vi "Ch_dis_to_Str_ADAM.vi"(4 "Ch Description":T1={"Ch Name"="", "Type"="", "Function"=enum."Analogue Input", "Ch State"=enum."On", "Calibration type"=enum."Raw", "A"=0.0, "B"=0.0, "C"=0.0, "D"=0.0, "Comments"="", "Address"={"Main"=0, "Ch."=0, "Sub"=0, "Port Name"=""}, "String"="", "Duty"=65535} {"Duty" format="%.0b"; "D" format="%#_5g"; "C" format="%#_5g"; "B" format="%#_5g"; "A" format="%#_5g"}) -> (1 "String Row":string)   [LabVIEW 2012]
uses:
  ADAM Controls/Ch_description_ADAM.ctl
  ADAM Controls/Module_type_ADAM.ctl
  ADAM Controls/Function_ADAM.ctl
  ADAM Controls/Channel_State.ctl
  ADAM Controls/Calib_type_ADAM.ctl
  ADAM Controls/Address.ctl
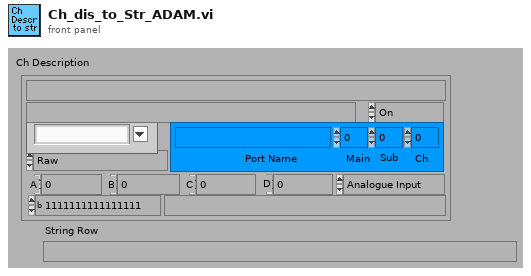
[diagram p1: front panel]
types:
  T1 = typedef "Ch_description_ADAM.ctl" = cluster{"Ch Name":string, "Type":T2, "Function":T3, "Ch State":T4, "Calibration type":T5, "A":dbl, "B":dbl, "C":dbl, "D":dbl, "Comments":string, "Address":T6, "String":string, "Duty":u16}
  T2 = typedef "Module_type_ADAM.ctl" = string
  T3 = typedef "Function_ADAM.ctl" = enum16{"Analogue Input", "Digital Input", "Event counter", "Event rate", "Analogue Output", "Digital Output", "Relay Output"}
  T4 = typedef "Channel_State.ctl" = enum16{"On", "Off", "Always On", "Always Off"}
  T5 = typedef "Calib_type_ADAM.ctl" = enum16{"Raw", "Bx + A", "Cx^2 + Bx + A", "Dx^3 + Cx^2 + Bx + A", "In Band", "Hi-Tec Q", "Hi-Tec M_dot", "Text"}
  T6 = typedef "Address.ctl" = cluster{"Main":i32, "Ch.":i32, "Sub":i32, "Port Name":string}
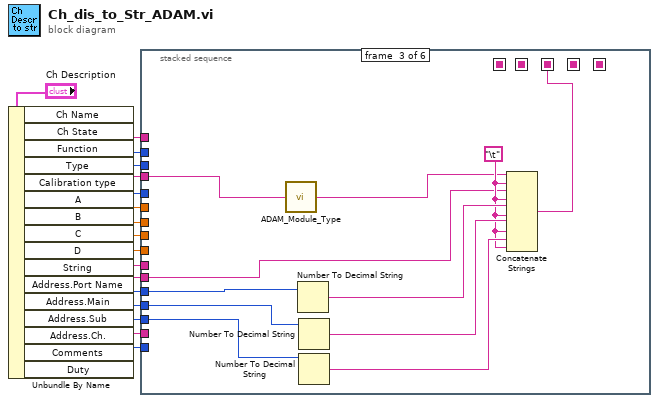
[diagram p0: block diagram]
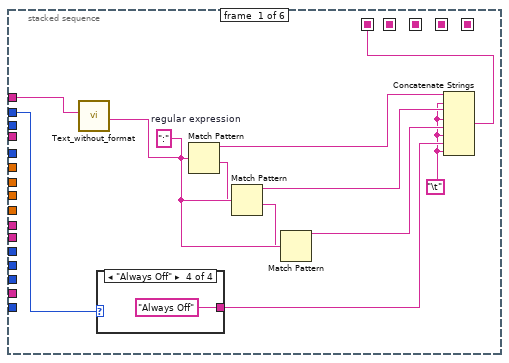
[diagram p2: hidden frame]
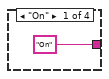
[diagram p3: hidden frame]
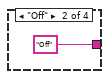
[diagram p4: hidden frame]
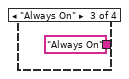
[diagram p5: hidden frame]
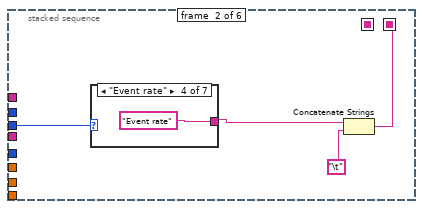
[diagram p6: hidden frame]
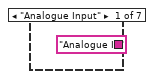
[diagram p7: hidden frame]
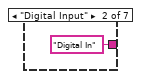
[diagram p8: hidden frame]
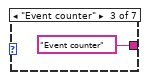
[diagram p9: hidden frame]
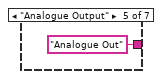
[diagram p10: hidden frame]
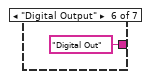
[diagram p11: hidden frame]
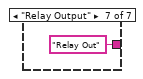
[diagram p12: hidden frame]
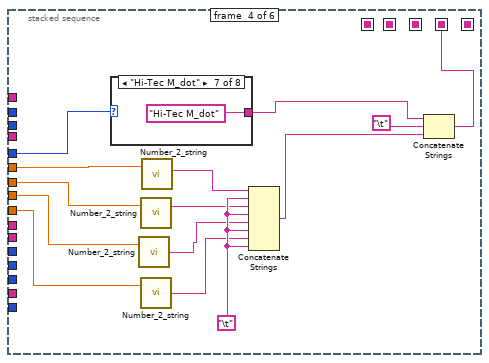
[diagram p13: hidden frame]
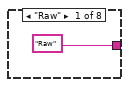
[diagram p14: hidden frame]
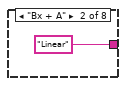
[diagram p15: hidden frame]
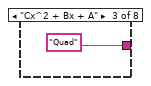
[diagram p16: hidden frame]
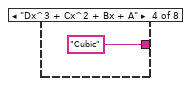
[diagram p17: hidden frame]
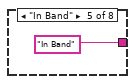
[diagram p18: hidden frame]
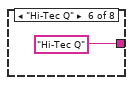
[diagram p19: hidden frame]
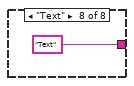
[diagram p20: hidden frame]
diagram:
  n1 = Unbundle By Name("Ch Description") -> ("Ch Name"=w7:string, "Ch State"=w9:T4, "Function"=w16:T3, "Type"=w15:T2, "Calibration type"=w14:T5, "A"=w13:dbl, "B"=w12:dbl, "C"=w10:dbl, "D"=w11:dbl, "String"=w8:string, "Address.Port Name"=w6:string, "Address.Main"=w5:i32, "Address.Sub"=w4:i32, "Address.Ch."=w3:i32, "Comments"=w2:string, "Duty"=w1:u16)
  n2 = stacked-sequence {
    seq-local: [_ _ w54 _ _ _] -> [_ _ _ _ _ w92]
    seq-local: [w23 _ _ _ _ _] -> [_ _ _ _ _ w89]
    seq-local: [_ _ _ w66 _ _] -> [_ _ _ _ _ w91]
    seq-local: [_ w34 _ _ _ _] -> [_ _ _ _ _ w88]
    seq-local: [_ _ _ _ w78 _] -> [_ _ _ _ _ w87]
    tunnel: w16 -> [_ w36 _ _ _ _]
    tunnel: w15 -> [_ _ w46 _ _ _]
    tunnel: w13 -> [_ _ _ w60 _ _]
    tunnel: w12 -> [_ _ _ w61 _ _]
    tunnel: w11 -> [_ _ _ w63 _ _]
    tunnel: w10 -> [_ _ _ w62 _ _]
    tunnel: w9 -> [w18 _ _ _ _ _]
    tunnel: w8 -> [_ _ _ _ w82 _]
    tunnel: w7 -> [w19 _ _ _ _ _]
    tunnel: w14 -> [_ _ _ w65 _ _]
    tunnel: w6 -> [_ _ w47 _ _ _]
    tunnel: w5 -> [_ _ w53 _ _ _]
    tunnel: w4 -> [_ _ w52 _ _ _]
    tunnel: w3 -> [_ _ w51 _ _ _]
    tunnel: w2 -> [_ _ _ _ w83 _]
    tunnel: w1 -> [_ _ _ _ _ w86]
    frame #0 {
      w28 = ":"  # regular expression
      w20 = "\t"
      n3 = call "Text_without_format.vi"("Input string"=w19) -> ("Output string"=w22:string)
      n4 = case shown="\"Always Off\"" w18 {
        tunnel: ["On" "Off" "Always On" "Always Off"] -> w21
        frame "On" {
        }
        frame "Off" {
        }
        frame "Always On" {
        }
        frame "Always Off" {
        }
      }
      n5 = Match Pattern(string=w22, regular expression=w28) -> (before substring=w29:string, after substring=w27:string)  [unwired: 3 out]
      n6 = Match Pattern(string=w27, regular expression=w28) -> (before substring=w25:string, after substring=w26:string)  [unwired: 3 out]
      n7 = Match Pattern(string=w26, regular expression=w28) -> (before substring=w24:string)  [unwired: 4 out]
      n8 = Concatenate Strings(w29, w20, w25, w20, w24, w20, w21, w20) -> (w23:string)
    }
    frame #1 {
      n9 = case shown="\"Event rate\"" w36 {
        tunnel: ["Analogue In" "Digital In" "Event counter" "Event rate" "Analogue Out" "Digital Out" "Relay Out"] -> w35
        frame "Analogue Input" {
        }
        frame "Digital Input" {
        }
        frame "Event counter" {
        }
        frame "Event rate" {
        }
        frame "Analogue Output" {
        }
        frame "Digital Output" {
        }
        frame "Relay Output" {
        }
      }
      n10 = Concatenate Strings(w35, "\t") -> (w34:string)
    }
    frame #2 {
      w48 = "\t"
      n11 = call "ADAM_Module_Type.vi"("Module Type"=w46) -> ("String"=w45:string)
      n12 = Number To Decimal String(number=w53) -> (decimal integer string=w55:string)  [unwired: 1 out]
      n13 = Number To Decimal String(number=w52) -> (decimal integer string=w50:string)  [unwired: 1 out]
      n14 = Number To Decimal String(number=w51) -> (decimal integer string=w49:string)  [unwired: 1 out]
      n15 = Concatenate Strings(w45, w48, w47, w48, w55, w48, w50, w48, w49, w48) -> (w54:string)
    }
    frame #3 {
      w67 = "\t"
      n16 = case shown="\"Hi-Tec M_dot\"" w65 {
        tunnel: ["Raw" "Linear" "Quad" "Cubic" "In Band" "Hi-Tec Q" "Hi-Tec M_dot" "Text"] -> w64
        frame "Raw" {
        }
        frame "Bx + A" {
        }
        frame "Cx^2 + Bx + A" {
        }
        frame "Dx^3 + Cx^2 + Bx + A" {
        }
        frame "In Band" {
        }
        frame "Hi-Tec Q" {
        }
        frame "Hi-Tec M_dot" {
        }
        frame "Text" {
        }
      }
      n17 = call "Number_2_string.vi"("number"=w62) -> ("String"=w57:string)  [unwired: 1 in]
      n18 = call "Number_2_string.vi"("number"=w61) -> ("String"=w58:string)  [unwired: 1 in]
      n19 = call "Number_2_string.vi"("number"=w63) -> ("String"=w56:string)  [unwired: 1 in]
      n20 = call "Number_2_string.vi"("number"=w60) -> ("String"=w59:string)  [unwired: 1 in]
      n21 = Concatenate Strings(w59, w67, w58, w67, w57, w67, w56, w67) -> (w69:string)
      n22 = Concatenate Strings(w64, "\t", w69) -> (w66:string)
    }
    frame #4 {
      n23 = call "Text_without_format.vi"("Input string"=w82) -> ("Output string"=w81:string)
      n24 = call "Text_without_format.vi"("Input string"=w83) -> ("Output string"=w80:string)
      n25 = Concatenate Strings(w81, "\t", w80) -> (w78:string)
    }
    frame #5 {
      n26 = Number To Decimal String(number=w86) -> (decimal integer string=w85:string)  [unwired: 1 out]
      n27 = Concatenate Strings(w89, w88, w92, w91, w87, "\t", w85) -> (→"String Row":string)
    }
  }
